vi "OriginSearch.vi"(8 "error in":errorcluster, 11 "VISA resource":refnum<visa-resource-name>) -> (0 "error out":errorcluster)   [LabVIEW 2014, in "GRBLMotionCore.lvlib"]
uses:
  <instrlib>/GRBL/GRBLMotionCore.lvlib
panel:
  out "Itration":i32
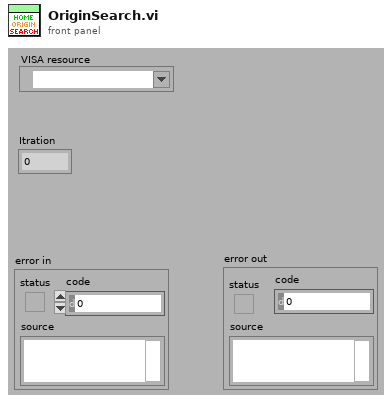
[diagram p1: front panel]
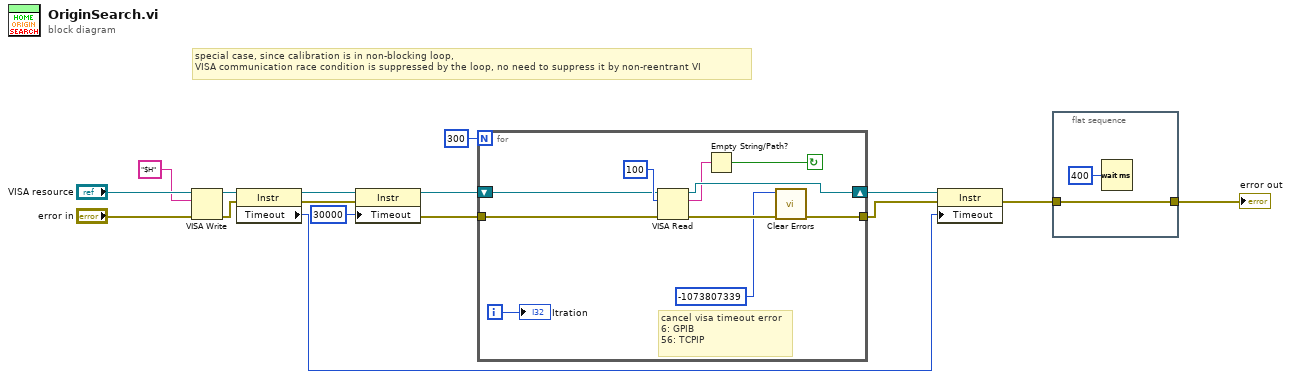
[diagram p0: block diagram]
diagram:
  # "special case, since calibration is in non-blocking loop,\nVISA communication race condition is suppressed by the loop, no need to suppress it by non-reentrant VI"
  n1 = VISA Write(VISA resource name="VISA resource", write buffer="$H", error in (no error)="error in") -> (VISA resource name out=w13:refnum<visa-resource-name>, error out=w10:errorcluster)  [unwired: 1 out]
  n2 = property class="Instr"(reference=w13, error in=w10) -> (reference out=w12:refnum<visa-resource-name>, error out=w9:errorcluster, "Timeout"=w6:u32)
  n3 = property class="Instr"(reference=w12, error in=w9, "Timeout"=u32 30000 ("General Settings:Timeout Value")) -> (reference out=w11:refnum<visa-resource-name>, error out=w8:errorcluster)
  n4 = for {
    N: 300 -> [_]
    tunnel: w8 -> [w19]
    tunnel: [w23] -> w4
    shift-right: [w24] -> w7
    shift-left: w11 -> [w18]
    i -> [w17]
    stop <- w20 continue-if-true
    # "cancel visa timeout error\n6: GPIB\n56: TCPIP"
    n5 = VISA Read(VISA resource name=w18, byte count=u32 100, error in (no error)=w19) -> (VISA resource name out=w24:refnum<visa-resource-name>, read buffer=w21:string, error out=w26:errorcluster)  [unwired: 1 out]
    n6 = Empty String/Path?(string/path=w21) -> (empty?=w20:bool)
    n7 = call <vilib>:"Clear Errors.vi"("error in (no error)"=w26, "specific error code to clear (0: all)"=-1073807339 ("[exception code]")) -> ("error out"=w23:errorcluster)  [unwired: 4 in, 1 out]
    "Itration" <- w17
  }
  n8 = property class="Instr"(reference=w7, error in=w4, "Timeout"=w6) -> (error out=w1:errorcluster)  [unwired: 1 out]
  n9 = flat-sequence {
    tunnel: [w27] -> w2
    tunnel: w1 -> [w27]
    frame #0 {
      n10 = Wait (ms)(milliseconds to wait=u32 400) -> ()  [unwired: 1 out]
    }
  }
  "error out" <- w2
